vi "Endpoint Configuration Page.vi"(8 "error in (no error)":errorcluster, 11 "Node Ptr":T4 format="%.0x") -> (0 "error out":errorcluster)   [LabVIEW 2017, in "SLSC Switch System Explorer.lvlib"]
uses:
  SLSC Switch System Explorer.lvlib
  <vilib>/NI Veristand/Custom Device API/Custom Device Item Ref.ctl
  Channel.ctl
  Channel Type.ctl
  Shared/UI Common/Sort Button.ctl
  Endpoint Configuration Page Controls.ctl
  16100924-b29d-4153-bcd0-e39b01036c8d.vi
  16100924-b29d-4153-bcd0-e39b01036c8d.vi/037e9b3c-b6e0-43a2-8d6b-c2c85ead1ecd.vi
  16100924-b29d-4153-bcd0-e39b01036c8d.vi/cbef740d-93e8-48c5-adb6-7f4ef73ad0ca.vi
  Shared/UI Common/Natural String Merge Sort.vi
  <vilib>/NI Veristand/Custom Device API/Custom Device API.lvlib
  Shared/UI Common/UI Common.lvlib
panel:
  in  "Sort":T1
  out "Configuration":string="Configuration"
  out "Endpoint":string="Endpoint"
  in  "Endpoints":T2[](array[typedef])
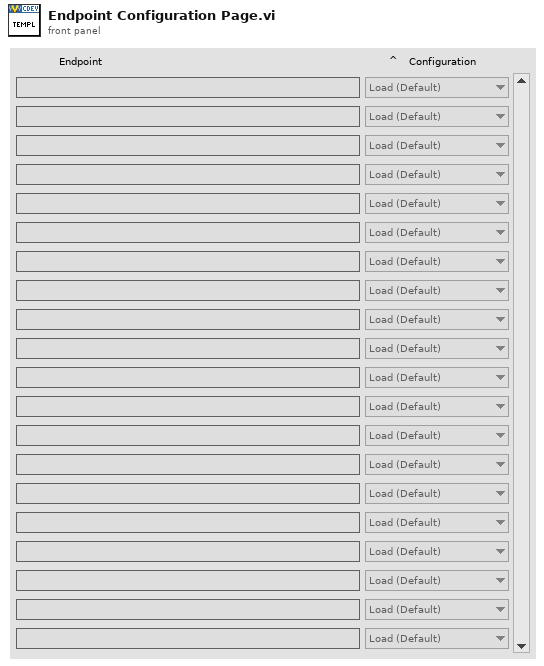
[diagram p1: front panel]
types:
  T1 = typedef "UI Common.lvlib/Sort Button.ctl" = bool
  T2 = typedef "SLSC Switch System Explorer.lvlib/Channel.ctl" = cluster{"Endpoint":string, "Configuration":T3}
  T3 = typedef "SLSC Switch System Explorer.lvlib/Channel Type.ctl" = enum16{"Load (Default)", "Source", "Configuration"}
  T4 = typedef "Custom Device API.lvlib/Custom Device Item Ref.ctl" = u64
  T5 = typedef "SLSC Switch System Explorer.lvlib/Endpoint Configuration Page Controls.ctl" = cluster{"Endpoints":refnum<vi>, "Endpoint Label":refnum<vi>, "Configuration Label":refnum<vi>, "Sort":refnum<vi>}
  T6 = typedef "Custom Device API.lvlib/Custom Device Commands.ctl" = enum16{"Default", "Item renamed", "Shutdown", "Dynamic button pressed"}
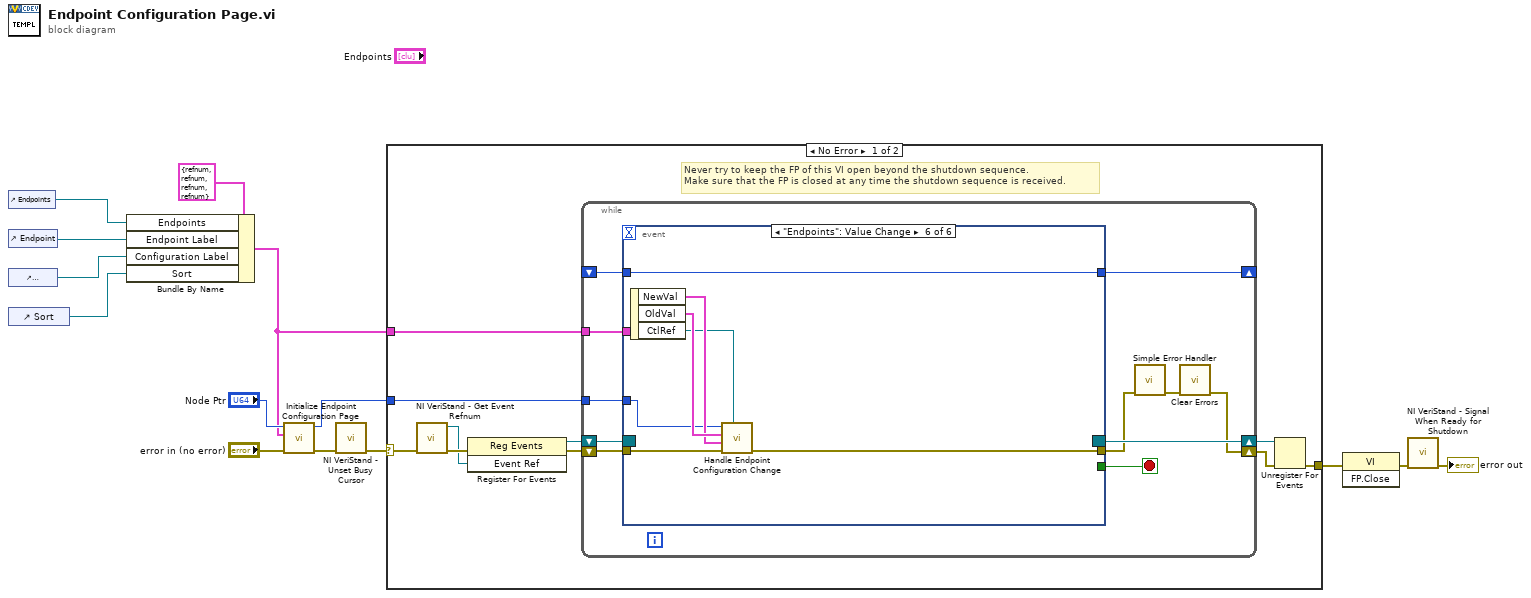
[diagram p0: block diagram]
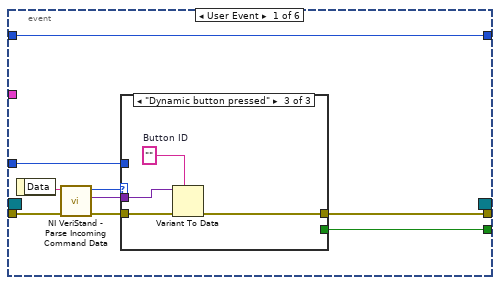
[diagram p2: hidden frame]
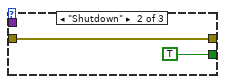
[diagram p4: hidden frame]
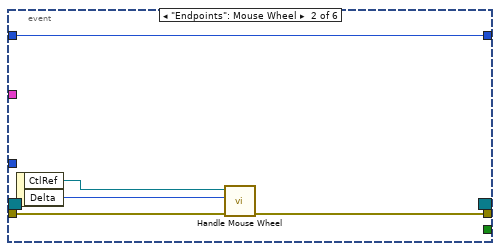
[diagram p5: hidden frame]
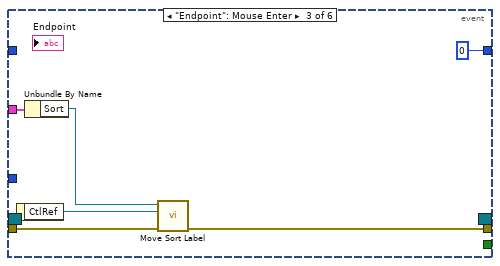
[diagram p6: hidden frame]
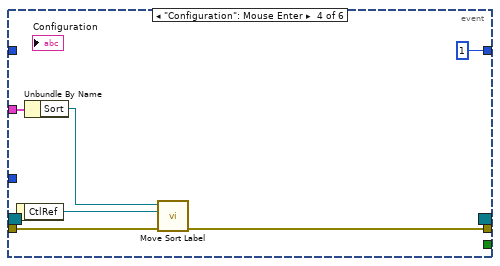
[diagram p7: hidden frame]
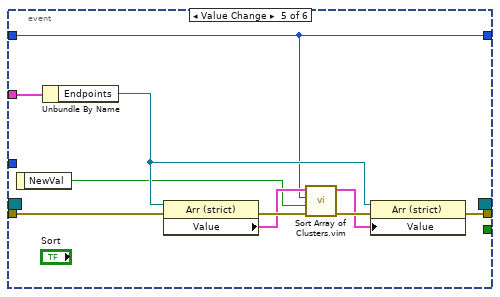
[diagram p8: hidden frame]
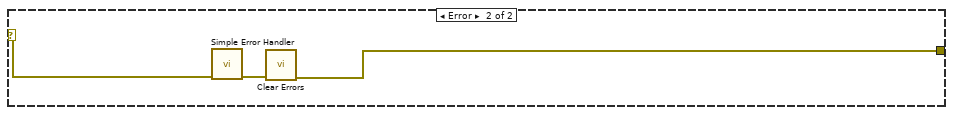
[diagram p9: hidden frame]
diagram:
  n1 = control-ref of="Endpoints"() -> (w7:refnum<vi>)
  n2 = control-ref of="Endpoint"() -> (w6:refnum<vi>)
  n3 = control-ref of="Configuration"() -> (w5:refnum<vi>)
  n4 = control-ref of="Sort"() -> (w4:refnum<vi>)
  n5 = Bundle By Name(cluster=T5 {"Endpoints"=refnum, "Endpoint Label"=refnum, "Configuration Label"=refnum, "Sort"=refnum} ("Endpoint Configuration Page Controls"), "Endpoints"=w7, "Endpoint Label"=w6, "Configuration Label"=w5, "Sort"=w4) -> (w3:T5)
  n6 = call "Initialize Endpoint Configuration Page.vi"("error in (no error)"="error in (no error)", "Endpoint Configuration Page Controls"=w3, "Node Ptr"="Node Ptr") -> ("error out"=w2:errorcluster, "Endpoint Configuration Section Ref out"=w9:T4)  [unwired: 7 in]
  n7 = call <vilib>:"NI VeriStand - Unset Busy Cursor.vi"("error in (no error)"=w2) -> ("error out"=w12:errorcluster)  [unwired: 10 out]
  n8 = case shown="No Error" w12 {
    selector: w12 -> [w19 w88]
    tunnel: [w22 w86] -> w14
    tunnel: w9 -> [w20 _]
    tunnel: w3 -> [w17 _]
    frame No Error {
      # "Never try to keep the FP of this VI open beyond the shutdown sequence.\nMake sure that the FP is closed at any time the shutdown sequence is received."
      n9 = call <vilib>:"NI VeriStand - Get Event Refnum.vi"("error in (no error)"=w19) -> ("error out"=w16:errorcluster, "Event Ref"=w15:refnum<user-event>)  [unwired: 9 out]
      n10 = register-events(error in=w16, w15) -> (reference out=w21:refnum<event-registration>, error out=w18:errorcluster)  [unwired: 1 in]
      n11 = while {
        tunnel: w20 -> [w31]
        shift-right: [w28] -> w23
        shift-left: w18 -> [w34]
        shift-right: [w35] -> w24
        shift-left: w21 -> [w33]
        shift-right: [w27] -> _
        shift-left: _ -> [w25]
        tunnel: w17 -> [w26]
        stop <- w32 stop-if-true
        n12 = event shown="[5] \"Endpoints\": Value Change" {
          selector: w33 -> [_ _ _ _ _ _]
          dyn-events: [_ _ _ _ _ _] -> w35
          timeout: _ -> [_ _ _ _ _ _]
          tunnel: w34 -> [w44 w56 w62 w68 w78 w84]
          tunnel: [w40 _ _ _ _ _] -> w32
          tunnel: [w39 w55 w61 w67 w73 w83] -> w30
          tunnel: w31 -> [w38 _ _ _ _ w79]
          tunnel: [w36 w53 0 ("index of element") 1 ("index of element") w69 w85] -> w27
          tunnel: w26 -> [_ _ w58 w64 w77 _]
          tunnel: w25 -> [w36 w53 _ _ w69 w85]
          event User Event {
            n13 = event-data() -> ("Data"=w43:string)  [unwired: 1 out]
            n14 = call <vilib>:"NI VeriStand - Parse Incoming Command Data.vi"("error in (no error)"=w44, "Incoming data"=w43) -> ("error out"=w42:errorcluster, "Outgoing data"=w37:variant, "Action"=w41:T6)  [unwired: 7 out]
            n15 = case shown="\"Dynamic button pressed\"" w41 {
              tunnel: w42 -> [w45 w46 w51]
              tunnel: [_ TRUE _] -> w40
              tunnel: [w45 w46 w48] -> w39
              tunnel: w38 -> [_ _ _]
              tunnel: w37 -> [_ _ w50]
              frame "Default", Default {
              }
              frame "Shutdown" {
              }
              frame "Dynamic button pressed" {
                w49 = ""  # Button ID
                n16 = Variant To Data(error in=w51, type=w49, Variant=w50) -> (error out=w48:errorcluster)  [unwired: 1 out]
              }
            }
          }
          event "Endpoints": Mouse Wheel {
            n17 = event-data() -> ("CtlRef"=w54:refnum<vi>, "Delta"=w52:i32)  [unwired: 1 out]
            n18 = call "Handle Mouse Wheel.vi"("error in (no error)"=w56, "delta"=w52, "Array Refnum"=w54) -> ("error out"=w55:errorcluster)  [unwired: 7 in, 1 out]
          }
          event "Endpoint": Mouse Enter {
            n19 = event-data() -> ("CtlRef"=w60:refnum<vi>)  [unwired: 1 out]
            n20 = Unbundle By Name(w58) -> ("Sort"=w57:refnum<vi>)
            n21 = call "Move Sort Label.vi"("error in (no error)"=w62, "Target Label"=w60, "Sort"=w57) -> ("error out"=w61:errorcluster)  [unwired: 8 in]
          }
          event "Configuration": Mouse Enter {
            n22 = event-data() -> ("CtlRef"=w66:refnum<vi>)  [unwired: 1 out]
            n23 = Unbundle By Name(w64) -> ("Sort"=w63:refnum<vi>)
            n24 = call "Move Sort Label.vi"("error in (no error)"=w68, "Target Label"=w66, "Sort"=w63) -> ("error out"=w67:errorcluster)  [unwired: 8 in]
          }
          event Value Change {
            n25 = event-data() -> ("NewVal"=w70:T1)  [unwired: 1 out]
            n26 = Unbundle By Name(w77) -> ("Endpoints"=w71:refnum<vi>)
            n27 = property class="Arr (strict)"(reference=w71, error in=w78) -> (error out=w76:errorcluster, "Value"=w75:T2[])  [unwired: 1 out]
            n28 = call "Sort Array of Clusters.vim"("error in (no error)"=w76, "Descending"=w70, "index"=w69, "Array"=w75) -> ("error out"=w74:errorcluster, "Sorted Array"=w72:T2[])  [unwired: 6 in]
            n29 = property class="Arr (strict)"(reference=w71, error in=w74, "Value"=w72) -> (error out=w73:errorcluster)  [unwired: 1 out]
          }
          event "Endpoints": Value Change {
            n30 = event-data() -> ("NewVal"=w81:T2[], "OldVal"=w82:T2[], "CtlRef"=w80:refnum<vi>)  [unwired: 1 out]
            n31 = call "Handle Endpoint Configuration Change.vi"("Array in"=w80, "error in (no error)"=w84, "NewVal"=w81, "OldVal"=w82, "Endpoint Configuration Section Ref in"=w79) -> ("error out"=w83:errorcluster)  [unwired: 5 in, 1 out]
          }
        }
        n32 = call <vilib>:"Simple Error Handler.vi"("error in (no error)"=w30) -> ("error out"=w29:errorcluster)  [unwired: 1 in, 7 out]
        n33 = call <vilib>:"Clear Errors.vi"("error in (no error)"=w29) -> ("error out"=w28:errorcluster)  [unwired: 1 in, 5 out]
      }
      n34 = Unregister For Events(event registration refnum=w24, error in=w23) -> (error out=w22:errorcluster)
    }
    frame Error {
      n35 = call <vilib>:"Simple Error Handler.vi"("error in (no error)"=w88) -> ("error out"=w87:errorcluster)  [unwired: 1 in, 7 out]
      n36 = call <vilib>:"Clear Errors.vi"("error in (no error)"=w87) -> ("error out"=w86:errorcluster)  [unwired: 1 in, 5 out]
    }
  }
  n37 = invoke class="VI" method="FP.Close"(error in=w14) -> (error out=w1:errorcluster)  [unwired: 2 in, 2 out]
  n38 = call <vilib>:"NI VeriStand - Signal When Ready for Shutdown.vi"("error in (no error)"=w1) -> ("error out"=→"error out":errorcluster)  [unwired: 10 out]
